vi "From Pad Values to Data Values.vi"(8 "Error In":errorcluster, 9 "button info":T1, 10 "axis info":T2, 11 "Calibration Cluster":T3) -> (0 "Error Out":errorcluster, 1 "Motor On":bool, 2 "Steering Wheel":i8(slide) min=-100 max=100 scale=-100.0..100.0, 3 "Speed":i8)   [LabVIEW 2014]
doc: "This VI converts from values on pad to values to send"
uses:
  Controls/Controllers Clusters/Game Pad Calibration Cluster.ctl
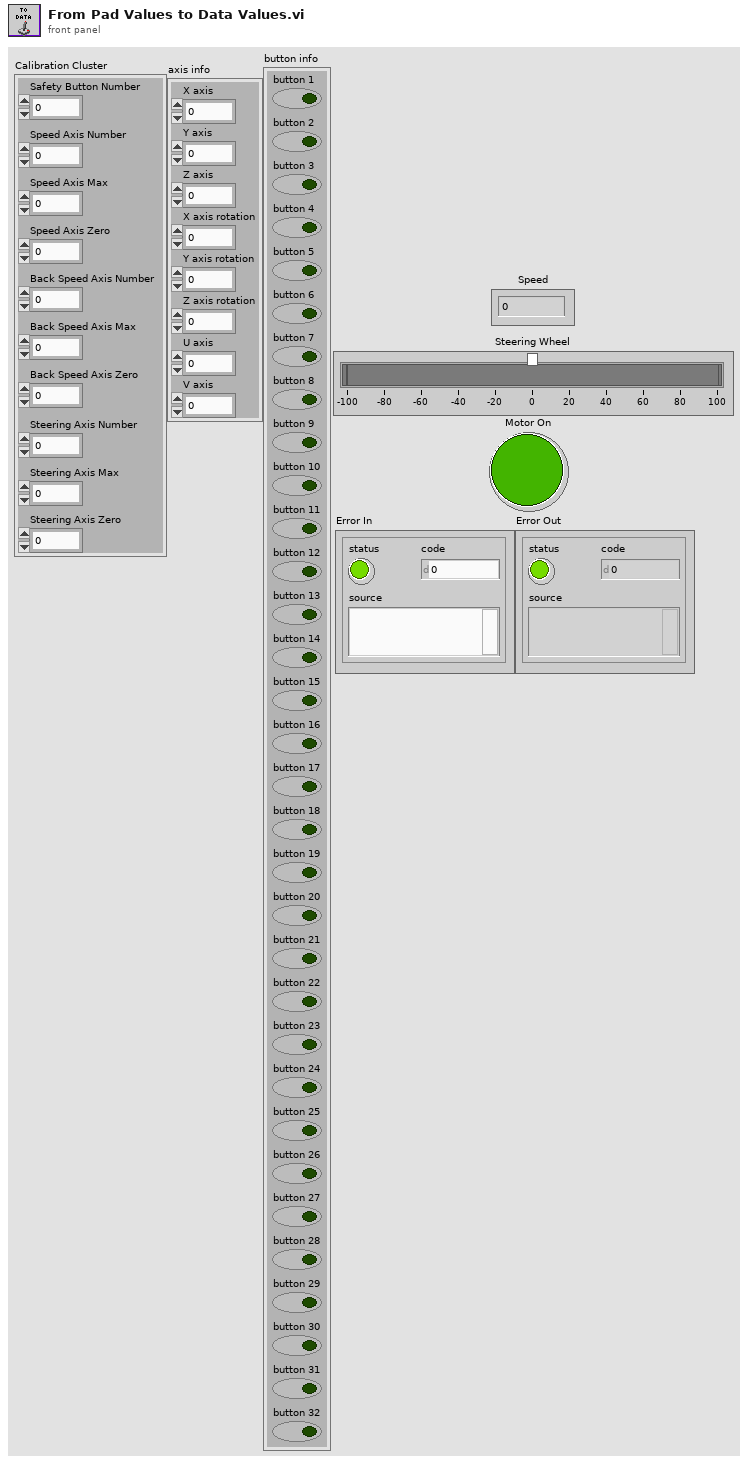
[diagram p1: front panel]
types:
  T1 = cluster{"button 1":bool, "button 2":bool, "button 3":bool, "button 4":bool, "button 5":bool, "button 6":bool, "button 7":bool, "button 8":bool, "button 9":bool, "button 10":bool, "button 11":bool, "button 12":bool, "button 13":bool, "button 14":bool, "button 15":bool, "button 16":bool, "button 17":bool, "button 18":bool, "button 19":bool, "button 20":bool, "button 21":bool, "button 22":bool, "button 23":bool, "button 24":bool, "button 25":bool, "button 26":bool, "button 27":bool, "button 28":bool, "button 29":bool, "button 30":bool, "button 31":bool, "button 32":bool}
  T2 = cluster{"X axis":i32, "Y axis":i32, "Z axis":i32, "X axis rotation":i32, "Y axis rotation":i32, "Z axis rotation":i32, "U axis":i32, "V axis":i32}
  T3 = typedef "Game Pad Calibration Cluster.ctl" = cluster{"Safety Button Number":u8, "Speed Axis Number":u8, "Speed Axis Max":i32, "Speed Axis Zero":i32, "Back Speed Axis Number":u8, "Back Speed Axis Max":i32, "Back Speed Axis Zero":i32, "Steering Axis Number":u8, "Steering Axis Max":i32, "Steering Axis Zero":i32}
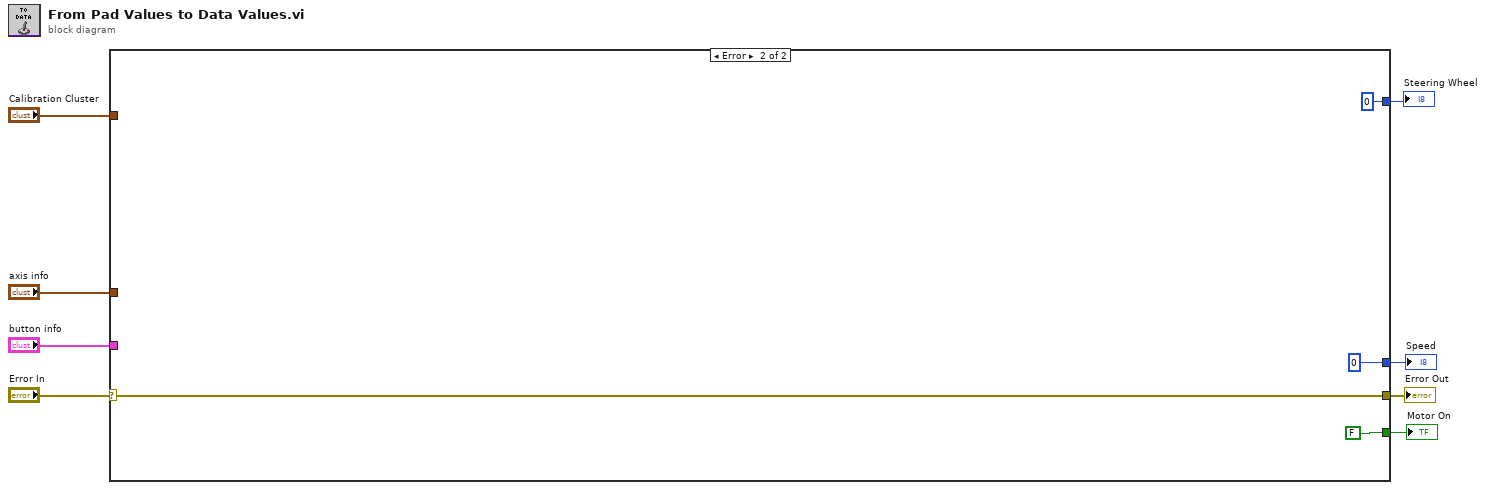
[diagram p0: block diagram]
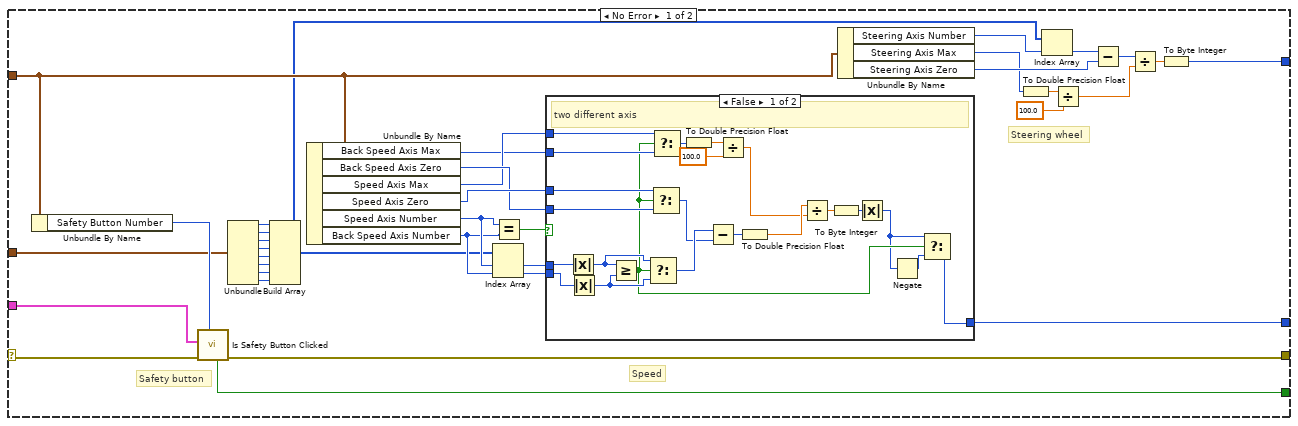
[diagram p2: hidden frame]
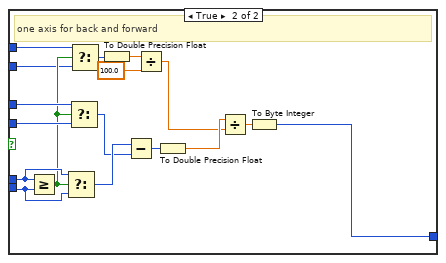
[diagram p3: hidden frame]
diagram:
  n1 = case shown="Error" "Error In" {
    selector: "Error In" -> [w44 w87]
    tunnel: [w41 w87] -> w7
    tunnel: "Calibration Cluster" -> [w20 _]
    tunnel: "axis info" -> [w39 _]
    tunnel: "button info" -> [w43 _]
    tunnel: [w40 FALSE ("Clicked?")] -> w3
    tunnel: [w21 i8 0] -> w2
    tunnel: [w9 i8 0] -> w1
    frame No Error {
      # "Steering wheel"
      # "Speed"
      # "Safety button"
      n2 = Unbundle By Name(w20) -> ("Safety Button Number"=w42:u8)
      n3 = call "Is Safety Button Clicked.vi"("Safety Button Number"=w42, "Error In"=w44, "Button Info"=w43) -> ("Error Out"=w41:errorcluster, "Clicked?"=w40:bool)  [unwired: 7 in]
      n4 = Unbundle(w39) -> ("X axis"=w38:i32, "Y axis"=w31:i32, "Z axis"=w32:i32, "X axis rotation"=w33:i32, "Y axis rotation"=w34:i32, "Z axis rotation"=w35:i32, "U axis"=w36:i32, "V axis"=w37:i32)
      n5 = Build Array(w38, w31, w32, w33, w34, w35, w36, w37) -> (w18:i32[])
      n6 = Unbundle By Name(w20) -> ("Back Speed Axis Max"=w22:i32, "Back Speed Axis Zero"=w24:i32, "Speed Axis Max"=w23:i32, "Speed Axis Zero"=w25:i32, "Speed Axis Number"=w30:u8, "Back Speed Axis Number"=w29:u8)
      n7 = Index Array(array=w18, index #1=w30, index #2=w29) -> (element #1=w27:i32, element #2=w26:i32)
      n8 = Equal?(x=w30, y=w29) -> (x = y?=w28:bool)
      n9 = case shown="False" w28 {
        tunnel: w27 -> [w52 w83]
        tunnel: w26 -> [w53 w82]
        tunnel: w25 -> [w55 w81]
        tunnel: w24 -> [w54 w80]
        tunnel: w23 -> [w57 w76]
        tunnel: w22 -> [w56 w75]
        tunnel: [w45 w67] -> w21
        frame False {
          # "two different axis"
          n10 = Absolute Value(x=w52) -> (abs(x)=w51:i32)
          n11 = Absolute Value(x=w53) -> (abs(x)=w50:i32)
          n12 = Greater Or Equal?(x=w51, y=w50) -> (x >= y?=w49:bool)
          n13 = Select(t=w51, s=w49, f=w50) -> (s? t:f=w66:i32)
          n14 = Select(t=w55, s=w49, f=w54) -> (s? t:f=w65:i32)
          n15 = Select(t=w57, s=w49, f=w56) -> (s? t:f=w64:i32)
          n16 = To Double Precision Float(number=w64) -> (double precision float=w63:dbl)
          n17 = Subtract(x=w66, y=w65) -> (x-y=w61:i32)
          n18 = Divide(x=w63, y=100.0) -> (x/y=w59:dbl)
          n19 = To Double Precision Float(number=w61) -> (double precision float=w60:dbl)
          n20 = Divide(x=w60, y=w59) -> (x/y=w58:dbl)
          n21 = To Byte Integer(number=w58) -> (8bit integer=w48:i8)
          n22 = Absolute Value(x=w48) -> (abs(x)=w46:i8)
          n23 = Negate(x=w46) -> (-x=w47:i8)
          n24 = Select(t=w46, s=w49, f=w47) -> (s? t:f=w45:i8)
        }
        frame True {
          # "one axis for back and forward"
          n25 = Greater Or Equal?(x=w83, y=w82) -> (x >= y?=w77:bool)
          n26 = Select(t=w83, s=w77, f=w82) -> (s? t:f=w79:i32)
          n27 = Select(t=w81, s=w77, f=w80) -> (s? t:f=w78:i32)
          n28 = Select(t=w76, s=w77, f=w75) -> (s? t:f=w74:i32)
          n29 = To Double Precision Float(number=w74) -> (double precision float=w73:dbl)
          n30 = Subtract(x=w79, y=w78) -> (x-y=w71:i32)
          n31 = Divide(x=w73, y=100.0) -> (x/y=w69:dbl)
          n32 = To Double Precision Float(number=w71) -> (double precision float=w70:dbl)
          n33 = Divide(x=w70, y=w69) -> (x/y=w68:dbl)
          n34 = To Byte Integer(number=w68) -> (8bit integer=w67:i8)
        }
      }
      n35 = Unbundle By Name(w20) -> ("Steering Axis Number"=w19:u8, "Steering Axis Max"=w15:i32, "Steering Axis Zero"=w16:i32)
      n36 = To Double Precision Float(number=w15) -> (double precision float=w14:dbl)
      n37 = Index Array(array=w18, index=w19) -> (element=w17:i32)
      n38 = Divide(x=w14, y=100.0) -> (x/y=w11:dbl)
      n39 = Subtract(x=w17, y=w16) -> (x-y=w12:i32)
      n40 = Divide(x=w12, y=w11) -> (x/y=w10:dbl)
      n41 = To Byte Integer(number=w10) -> (8bit integer=w9:i8)
    }
    frame Error {
    }
  }
  "Error Out" <- w7
  "Speed" <- w2
  "Steering Wheel" <- w1
  "Motor On" <- w3
